vi "LSTM-generic-function.vi"(0 "piecewise function":dbl[][](array[numeric]), 5 "h":T1, 7 "x":T1, 8 "b":T1, 9 "U":T1, 10 "W":T1) -> (2 "y":T1)   [LabVIEW 2020]
uses:
  <vilib>/Analysis/Matrix/Datatypes/RealMatrix.ctl
  <vilib>/Analysis/baseanly.llb/Real A x B.vi
  <vilib>/Analysis/Matrix/Numeric/Add/Add - RM,RM.vi
  <vilib>/Analysis/Matrix/NI_Matrix.lvlib
  <vilib>/Analysis/NI_AALBase.lvlib
panel:
  out "indicator 2":T1
  out "indicator":T1
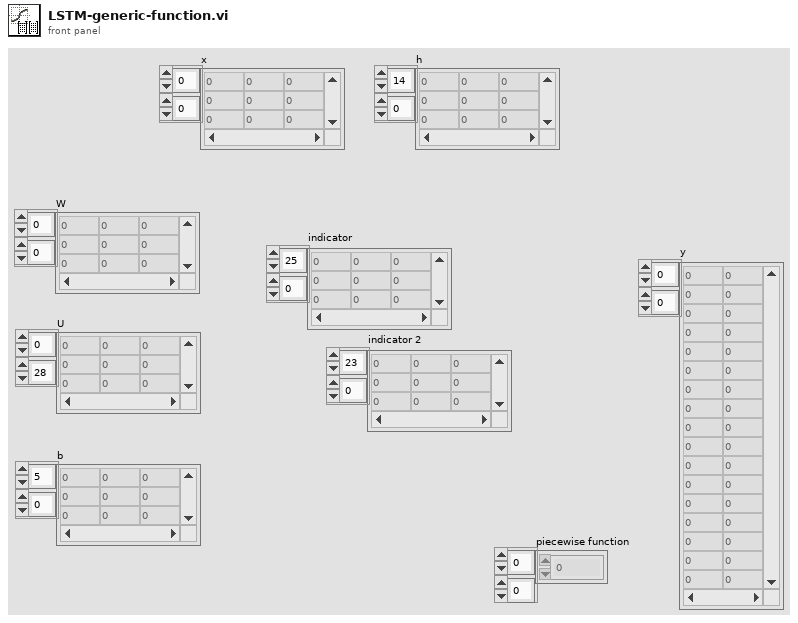
[diagram p1: front panel]
types:
  T1 = typedef "NI_Matrix.lvlib/RealMatrix.ctl" = dbl[][]
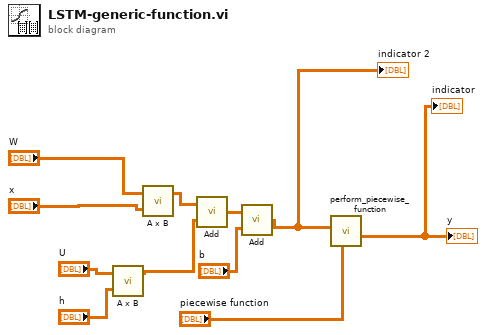
[diagram p0: block diagram]
diagram:
  n1 = call-poly <vilib>:"A x B.vi"("B"="h", "A"="U") -> ("A x B"=w6:T1)  [unwired: 1 out]
  n2 = call-poly <vilib>:"A x B.vi"("B"="x", "A"="W") -> ("A x B"=w3:T1)  [unwired: 1 out]
  n3 = call-poly <vilib>:"Add.vi"("Real Matrix B"=w6, "Real Matrix A"=w3) -> ("A + B"=w9:T1)
  n4 = call-poly <vilib>:"Add.vi"("Real Matrix B"="b", "Real Matrix A"=w9) -> ("A + B"=w1:T1)
  "indicator 2" <- w1
  n5 = call "perform_piecewise_function.vi"("function array"="piecewise function", "x"=w1) -> ("y"=→"y" →"indicator":T1)  [unwired: 9 in]
